vi "Write Modbus Enqueuer.vi"(8 "error in (no error)":errorcluster, 10 "Actor Framework:Message Enqueuer":refnum<class "Message Enqueuer.lvclass">, 11 "Algorythm in":refnum<class "Algorythm.lvclass">) -> (0 "error out":errorcluster, 3 "Algorythm out":refnum<class "Algorythm.lvclass">)   [LabVIEW 2020, in "Algorythm.lvlib" / "Algorythm.lvclass"]
uses:
  Algorythm.lvclass
  <vilib>/ActorFramework/Message Enqueuer/Message Enqueuer.lvclass
  Algorythm.lvclass/Algorythm.ctl
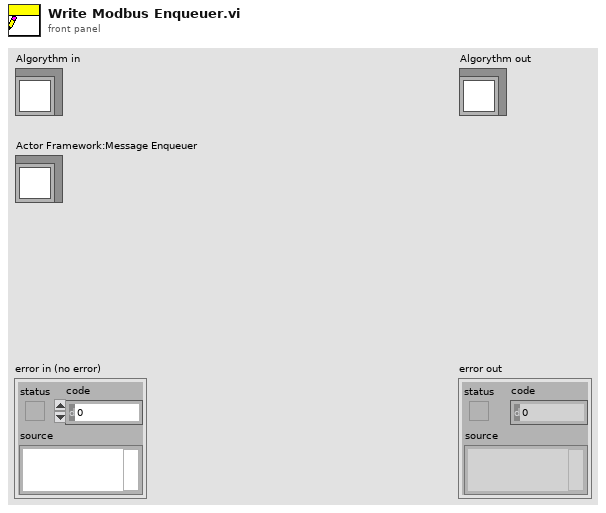
[diagram p1: front panel]
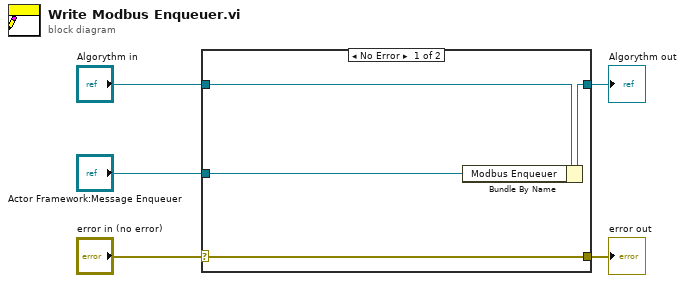
[diagram p0: block diagram]
diagram:
  n1 = case shown="No Error" "error in (no error)" {
    selector: "error in (no error)" -> [w9 w10]
    tunnel: [w9 w10] -> w4
    tunnel: [w7 w11] -> w2
    tunnel: "Algorythm in" -> [w8 w11]
    tunnel: "Actor Framework:Message Enqueuer" -> [w6 _]
    frame No Error {
      n2 = Bundle By Name(cluster=w8, "Modbus Enqueuer"=w6) -> (w7:refnum<class "Algorythm.lvclass">)
    }
    frame Error {
    }
  }
  "error out" <- w4
  "Algorythm out" <- w2
